vi "Auto Loop 2.vi"(2 "Auto State":u8, 3 "Call Context":T3) -> (0 "Loop 2 Data":T1, 1 "SubState 2":T2)   [LabVIEW 2013]
uses:
  <vilib>/Rock Robotics/WPI/DriverStation/WPI_DriverStationDerivedRobotMode.ctl
  typedefs/subStates.ctl
  typedefs/Loop Datatypes/Loop 2 Datatype.ctl
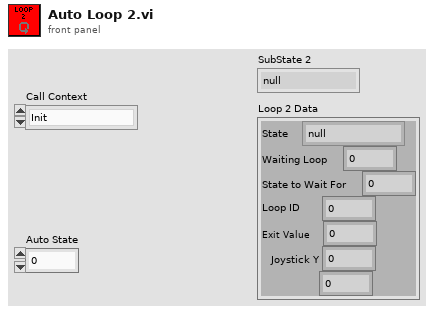
[diagram p1: front panel]
types:
  T1 = typedef "Loop 2 Datatype.ctl" = cluster{"State":T2, "Waiting Loop":i32, "State to Wait For":i32, "Loop ID":i32, "Exit Value":i32, "Joystick Y":dbl, "Joystick Z":dbl}
  T2 = typedef "subStates.ctl" = enum16{"null", "wait", "driver control", "auto", "manual override", "hold position", "rotate", "pickup", "pass", "load", "goto shoot", "shoot high goal", "shoot low goal", "cancel arm", "cancel shooter", "end"}
  T3 = typedef "WPI_DriverStationDerivedRobotMode.ctl" = enum16{"Init", "Execute", "Stop"}
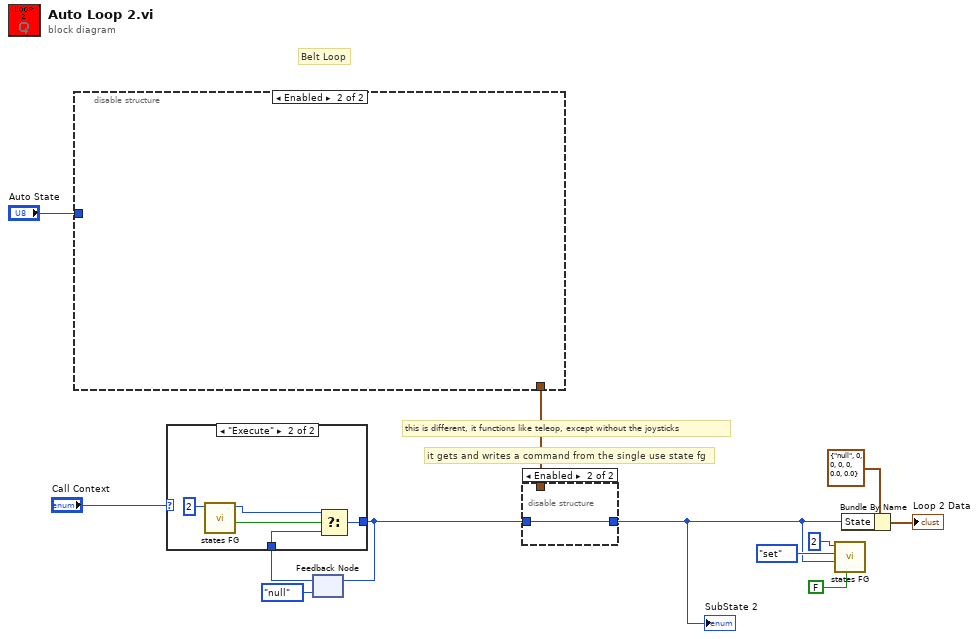
[diagram p0: block diagram]
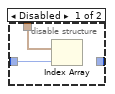
[diagram p2: hidden frame]
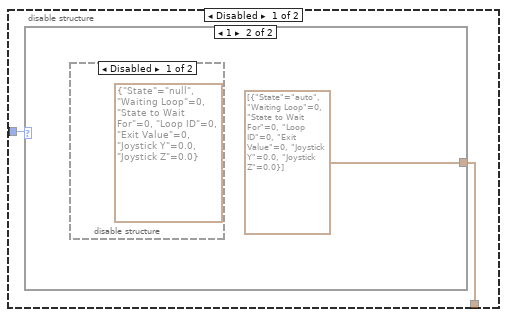
[diagram p3: hidden frame]
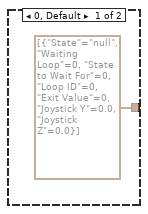
[diagram p4: hidden frame]
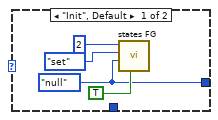
[diagram p6: hidden frame]
diagram:
  # "Belt Loop"
  # "it gets and writes a command from the single use state fg"
  # "this is different, it functions like teleop, except without the joysticks"
  n1 = disable-structure shown="Enabled" {
    disable-tunnel: "Auto State" -> [w14 _]
    disable-tunnel: [w13 _] -> w9
    frame Disabled {
      n2 = case shown="1" w14 {
        tunnel: [T1[] [{"State"=enum."null", "Waiting Loop"=0, "State to Wait For"=0, "Loop ID"=0, "Exit Value"=0, "Joystick Y"=0.0, "Joystick Z"=0.0}] T1[] [{"State"=enum."auto", "Waiting Loop"=0, "State to Wait For"=0, "Loop ID"=0, "Exit Value"=0, "Joystick Y"=0.0, "Joystick Z"=0.0}]] -> w13
        frame 0, Default {
        }
        frame 1 {
          n3 = disable-structure shown="Disabled" {
            frame Disabled {
              (unwired) T1 {"State"=enum."null", "Waiting Loop"=0, "State to Wait For"=0, "Loop ID"=0, "Exit Value"=0, "Joystick Y"=0.0, "Joystick Z"=0.0} ("Loop 2 Data")
            }
            frame Enabled {
            }
          }
        }
      }
    }
    frame Enabled {
    }
  }
  n4 = feedback #1(subStates."null" ("subState out")) -> (w10:T2)
  n5 = case shown="\"Execute\"" "Call Context" {
    tunnel: w10 -> [_ w24]
    tunnel: [w17 w23] -> w8
    frame "Init", Default {
      w17 = subStates."null" ("subState in")
      n6 = call "states FG.vi"("exit in"=TRUE, "subState in"=w17, "menu (get)"=enum16{"set", "get"}."set", "Loop ID"=2) -> ()  [unwired: 4 in, 4 out]
    }
    frame "Execute" {
      n7 = call "states FG.vi"("Loop ID"=2) -> ("exit out"=w22:bool, "subState out"=w21:T2)  [unwired: 7 in, 2 out]
      n8 = Select(t=w21, s=w22, f=w24) -> (s? t:f=w23:T2)
    }
  }
  n9 = feedback-in #1(w8) -> ()
  n10 = disable-structure shown="Enabled" {
    disable-tunnel: w9 -> [w27 _]
    disable-tunnel: w8 -> [w26 w28]
    disable-tunnel: [_ w28] -> w1
    frame Disabled {
      n11 = Index Array(array=w27, index=w26) -> ()  [unwired: 1 out]
    }
    frame Enabled {
    }
  }
  "SubState 2" <- w1
  n12 = call "states FG.vi"("exit in"=FALSE, "subState in"=w1, "menu (get)"=enum16{"set", "get"}."set", "Loop ID"=2) -> ()  [unwired: 4 in, 4 out]
  n13 = Bundle By Name(cluster=T1 {"State"=enum."null", "Waiting Loop"=0, "State to Wait For"=0, "Loop ID"=0, "Exit Value"=0, "Joystick Y"=0.0, "Joystick Z"=0.0} ("Loop 2 Data"), "State"=w1) -> (→"Loop 2 Data":T1)
